vi "CRC_add.vi"(8 "error in (no error)":errorcluster, 11 "ISO 14443 A DOWN in":refnum<class "ISO 14443 A DOWN.lvclass">) -> (0 "error out":errorcluster, 3 "ISO 14443 A DOWN out":refnum<class "ISO 14443 A DOWN.lvclass">)   [LabVIEW 2019, in "ISO 14443 A DOWN.lvclass"]
uses:
  ISO 14443 A DOWN.lvclass
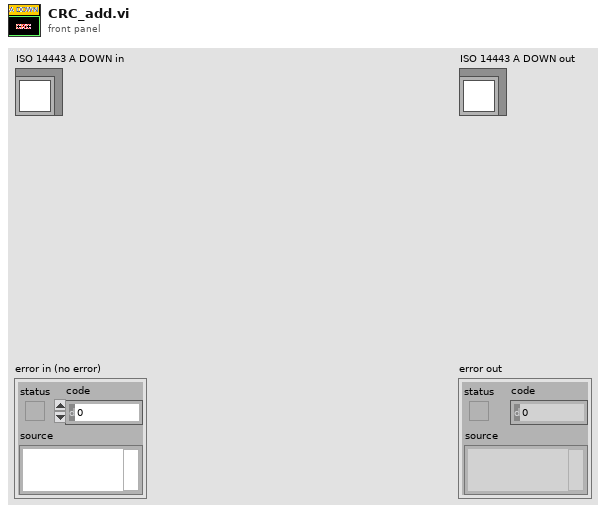
[diagram p1: front panel]
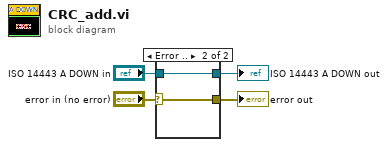
[diagram p0: block diagram]
diagram:
  n1 = case shown="Error .." "error in (no error)" {
    selector: "error in (no error)" -> [w6 w7]
    tunnel: [w6 w7] -> w3
    tunnel: "ISO 14443 A DOWN in" -> [w5 w8]
    tunnel: [w5 w8] -> w1
    frame No Error {
    }
    frame Error {
    }
  }
  "error out" <- w3
  "ISO 14443 A DOWN out" <- w1
